vi "Facade.vi"(0 "Data In":T5, 2 "Display State In":T2={"logTable"=refnum, "max items"=500, "displaydata"=[], "data"=[], "Auto Scroll"=TRUE, "current item"=500, "col headers"=[], "Add to Top"=TRUE, "Auto resize"=TRUE, "col size"=[], "filters"=[], "color cells"=[]}, 3 "Container State":T4) -> (6 "Data Out":T5, 7 "Display State Out":T2={"logTable"=refnum, "max items"=500, "displaydata"=[], "data"=[], "Auto Scroll"=TRUE, "current item"=500, "col headers"=[], "Add to Top"=TRUE, "Auto resize"=TRUE, "col size"=[], "filters"=[], "color cells"=[]}, 8 "Action":T1)   [LabVIEW 2017, in "UI-DisplayTable(dev).xctl"]
uses:
  UI-DisplayTable(dev).xctl
  Data.ctl
  <vilib>/_xctls/Container State.ctl
  State.ctl
  Support/DEF-Filter.ctl
  <vilib>/_xctls/Action.ctl
  <vilib>/_xctls/XControlSupport.lvlib
panel:
  out "logTable":string[][](table)
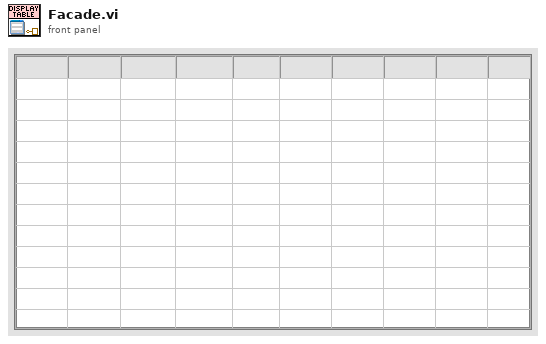
[diagram p1: front panel]
types:
  T1 = typedef "XControlSupport.lvlib/Action.ctl" = cluster{"Data Changed?":bool, "State Changed?":bool, "Action Name":string}
  T2 = typedef "UI-DisplayTable(dev).xctl/State.ctl" = cluster{"logTable":refnum<vi>, "max items":i32, "displaydata":string[][], "data":string[][], "Auto Scroll":bool, "current item":i32, "col headers":string[], "Add to Top":bool, "Auto resize":bool, "col size":i32[], "filters":T3[], "color cells":cluster{"color cell":cluster{"Column":string, "Value":string, "Highlight Column":string}, "Color Box":u32}[]}
  T3 = typedef "UI-DisplayTable(dev).xctl/DEF-Filter.ctl" = cluster{"column":string, "value":string[]}
  T4 = typedef "XControlSupport.lvlib/Container State.ctl" = cluster{"Indicator?":bool, "Run Mode?":bool, " Refnum":refnum<vi>}
  T5 = typedef "UI-DisplayTable(dev).xctl/Data.ctl" = i32
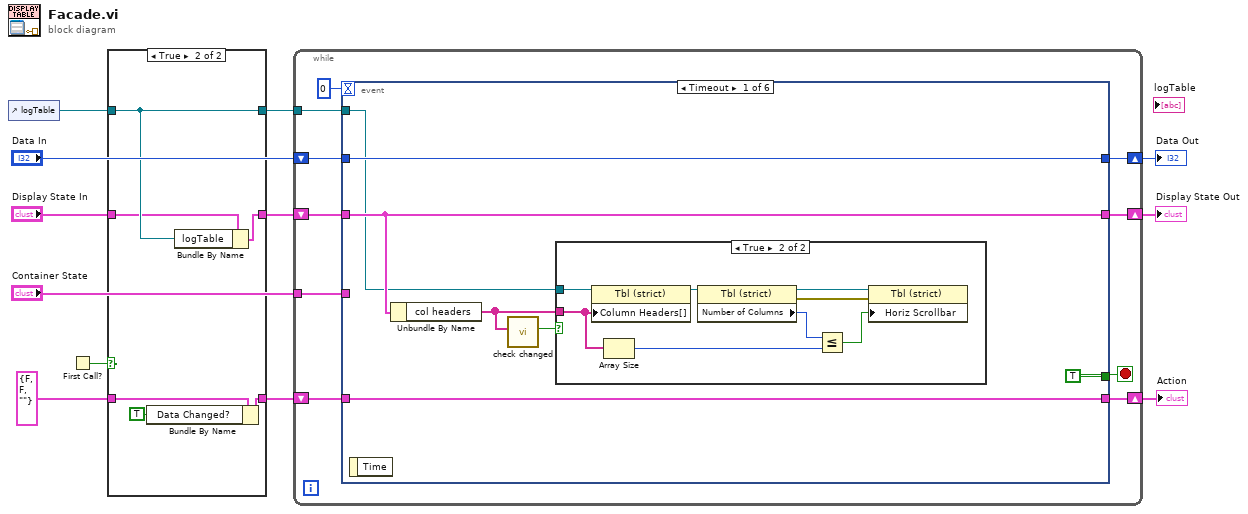
[diagram p0: block diagram]
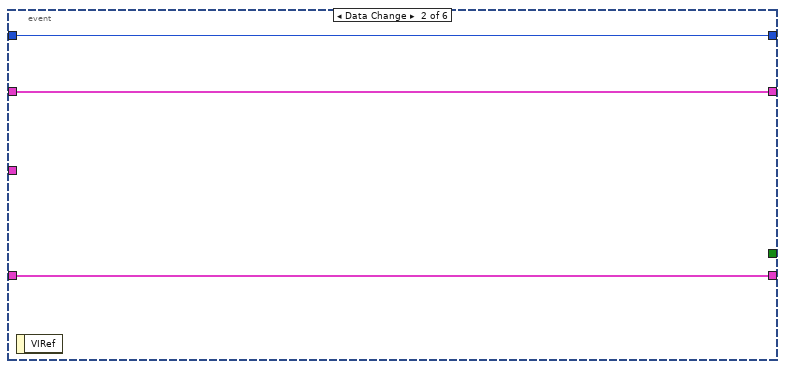
[diagram p4: hidden frame]
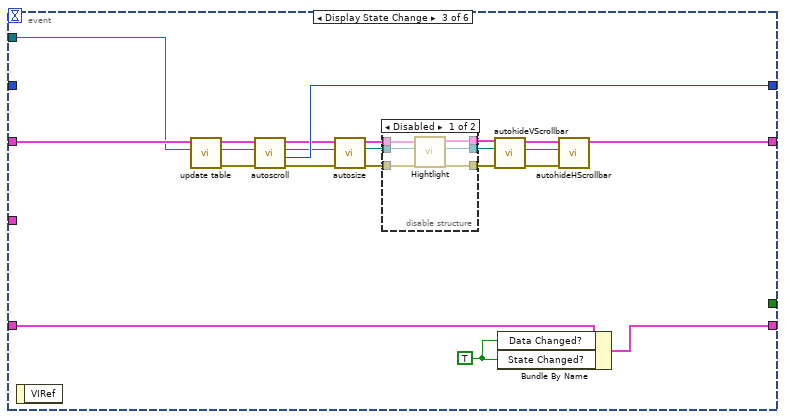
[diagram p5: hidden frame]
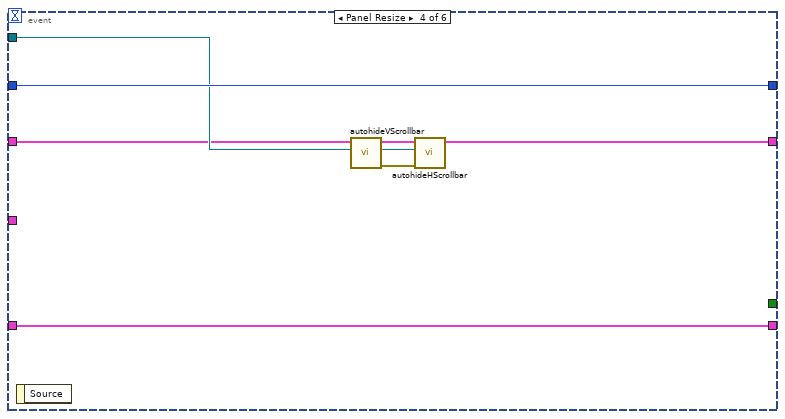
[diagram p7: hidden frame]
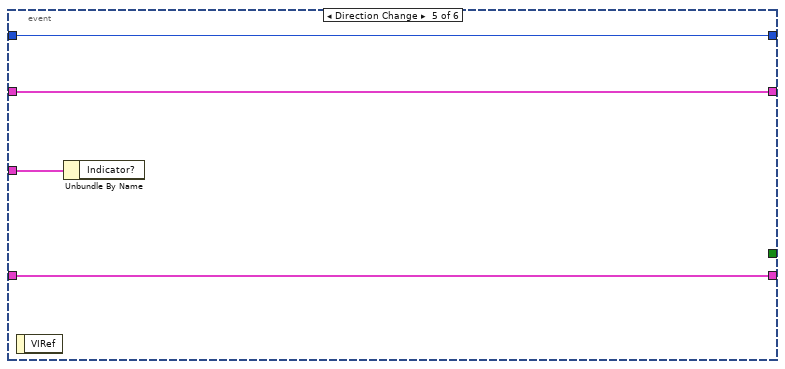
[diagram p8: hidden frame]
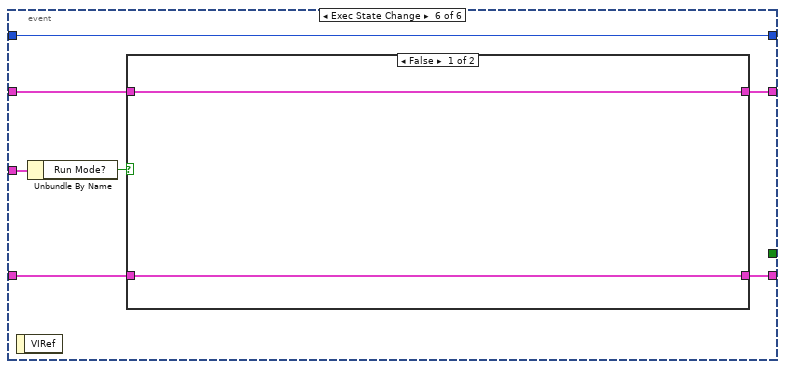
[diagram p9: hidden frame]
diagram:
  n1 = control-ref of="logTable"() -> (w6:refnum<vi>)
  n2 = First Call?() -> (First Call?: T/F=w1:bool)
  n3 = case shown="True" w1 {
    tunnel: [w15 w20] -> w7
    tunnel: w6 -> [w15 w20]
    tunnel: [w14 w21] -> w5
    tunnel: "Display State In" -> [w14 w19]
    tunnel: [w13 w17] -> w3
    tunnel: T1 {"Data Changed?"=FALSE, "State Changed?"=FALSE, "Action Name"=""} ("Action") -> [w13 w18]
    frame False {
    }
    frame True {
      n4 = Bundle By Name(cluster=w18, "Data Changed?"=TRUE) -> (w17:T1)
      n5 = Bundle By Name(cluster=w19, "logTable"=w20) -> (w21:T2)
    }
  }
  n6 = while {
    shift-right: [w30] -> w9
    shift-left: w5 -> [w31]
    tunnel: "Container State" -> [w27]
    shift-right: [w25] -> w12
    shift-left: "Data In" -> [w26]
    shift-right: [w23] -> w8
    shift-left: w3 -> [w24]
    tunnel: w7 -> [w22]
    stop <- w29 stop-if-true
    n7 = event shown="[0] Timeout" {
      selector: _ -> [_ _ _ _ _ _]
      dyn-events: _ -> [_ _ _ _ _ _]
      timeout: 0 -> [_ _ _ _ _ _]
      tunnel: w31 -> [w35 w48 w68 w83 w91 w96]
      tunnel: [w35 w48 w58 w82 w91 w95] -> w30
      tunnel: [TRUE _ _ _ _ _] -> w29
      tunnel: w27 -> [_ _ _ _ w92 w99]
      tunnel: w26 -> [w36 w49 _ w88 w90 w98]
      tunnel: [w36 w49 w63 w88 w90 w98] -> w25
      tunnel: [w37 w47 w70 w87 w89 w94] -> w23
      tunnel: w24 -> [w37 w47 w71 w87 w89 w93]
      tunnel: w22 -> [w32 _ w65 w86 _ _]
      event Timeout {
        n8 = event-data() -> ()  [unwired: 1 in, 1 out]
        n9 = Unbundle By Name(w35) -> ("col headers"=w33:string[])
        n10 = call "check changed.vi"("data"=w33) -> ("changed?"=w34:bool)  [unwired: 9 in, 1 out]
        n11 = case shown="True" w34 {
          tunnel: w33 -> [_ w44]
          tunnel: w32 -> [_ w46]
          frame False {
          }
          frame True {
            n12 = property class="Tbl (strict)"(reference=w46, "Column Headers[]"=w44) -> (reference out=w45:refnum<vi>)  [unwired: 1 in, 1 out]
            n13 = Array Size(array=w44) -> (size(s)=w39:i32)
            n14 = property class="Tbl (strict)"(reference=w45) -> (reference out=w43:refnum<vi>, error out=w42:errorcluster, "Number of Columns"=w41:u32)  [unwired: 1 in]
            n15 = Less Or Equal?(x=w41, y=w39) -> (x <= y?=w40:bool)
            n16 = property class="Tbl (strict)"(reference=w43, error in=w42, "Horiz Scrollbar"=w40) -> ()  [unwired: 2 out]
          }
        }
      }
      event Data Change {
        n17 = event-data() -> ()  [unwired: 1 in, 1 out]
      }
      event Display State Change {
        w69 = TRUE ("State Changed?")
        n18 = event-data() -> ()  [unwired: 1 in, 1 out]
        n19 = call "update table.vi"("Table in"=w65, "State"=w68) -> ("error out"=w64:errorcluster, "Table out"=w66:refnum<vi>, "State (dup)"=w67:T2)  [unwired: 7 in]
        n20 = call "autoscroll.vi"("error in (no error)"=w64, "Table in"=w66, "State"=w67) -> ("error out"=w56:errorcluster, "Number of Rows"=w63:i32, "Table out"=w61:refnum<vi>, "State (dup)"=w62:T2)  [unwired: 5 in]
        n21 = call "autosize.vi"("error in (no error)"=w56, "Table in"=w61, "State"=w62) -> ("error out"=w55:errorcluster, "Table out"=w54:refnum<vi>, "State (dup)"=w53:T2)  [unwired: 6 in]
        n22 = disable-structure shown="Disabled" {
          disable-tunnel: w55 -> [w77 w78]
          disable-tunnel: w54 -> [w76 w79]
          disable-tunnel: w53 -> [w75 w80]
          disable-tunnel: [w74 w80] -> w52
          disable-tunnel: [w73 w79] -> w51
          disable-tunnel: [w72 w78] -> w50
          frame Disabled {
            n23 = call "Hightlight.vi"("error in (no error)"=w77, "Table in"=w76, "State"=w75) -> ("error out"=w72:errorcluster, "Table out"=w73:refnum<vi>, "State (dup)"=w74:T2)  [unwired: 6 in]
          }
          frame Enabled {
          }
        }
        n24 = call "autohideVScrollbar.vi"("error in (no error)"=w50, "Table in"=w51, "State"=w52) -> ("error out"=w57:errorcluster, "Table out"=w59:refnum<vi>, "State (dup)"=w60:T2)  [unwired: 6 in]
        n25 = Bundle By Name(cluster=w71, "Data Changed?"=w69, "State Changed?"=w69) -> (w70:T1)
        n26 = call "autohideHScrollbar.vi"("error in (no error)"=w57, "Table in"=w59, "State"=w60) -> ("State (dup)"=w58:T2)  [unwired: 6 in, 2 out]
      }
      event Panel Resize {
        n27 = event-data() -> ()  [unwired: 1 in, 1 out]
        n28 = call "autohideVScrollbar.vi"("Table in"=w86, "State"=w83) -> ("error out"=w81:errorcluster, "Table out"=w85:refnum<vi>, "State (dup)"=w84:T2)  [unwired: 7 in]
        n29 = call "autohideHScrollbar.vi"("error in (no error)"=w81, "Table in"=w85, "State"=w84) -> ("State (dup)"=w82:T2)  [unwired: 6 in, 2 out]
      }
      event Direction Change {
        n30 = event-data() -> ()  [unwired: 1 in, 1 out]
        n31 = Unbundle By Name(w92) -> ()  [unwired: 1 out]
      }
      event Exec State Change {
        n32 = event-data() -> ()  [unwired: 1 in, 1 out]
        n33 = Unbundle By Name(w99) -> ("Run Mode?"=w97:bool)
        n34 = case shown="False" w97 {
          tunnel: w96 -> [w101 w103]
          tunnel: [w101 w103] -> w95
          tunnel: [w100 w102] -> w94
          tunnel: w93 -> [w100 w102]
          frame False {
          }
          frame True {
          }
        }
      }
    }
  }
  "Display State Out" <- w9
  "Data Out" <- w12
  "Action" <- w8
